vi "Delete.vi"(5 "Delete all found":bool, 6 "$Path or Item Name":string, 7 "error in (no error)":errorcluster, 9 "Offset":i32, 10 "JSON":string="{}") -> (0 "error out":errorcluster, 1 "<JSON> First Deleted Item":string, 2 "Number Deleted":i32, 3 "<JSON>":string caption="<JSON>With Item Deleted")   [LabVIEW 2021, in "json.facade.lvlib"]
doc: "Deletes JSON item at the JSON Path specified. If \"Delete all found\" is True, will delete all items matching the path. Else will just delete the first found."
uses:
  json.facade.lvlib
  jsontext/JSONtext.lvlib
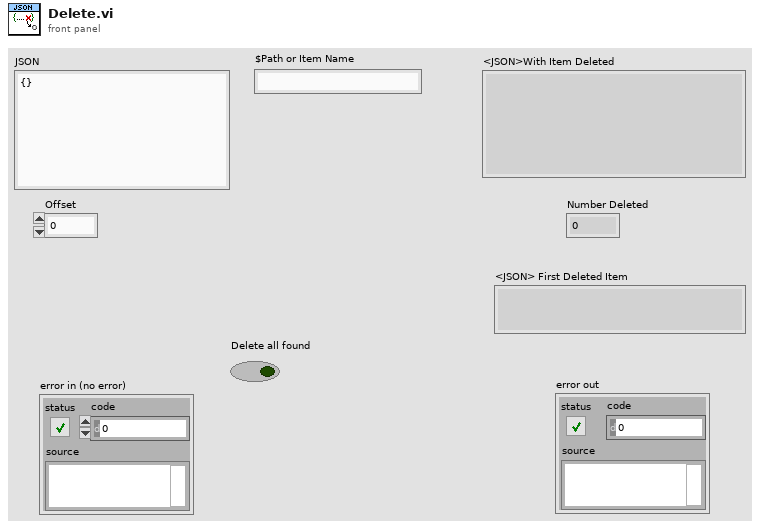
[diagram p1: front panel]
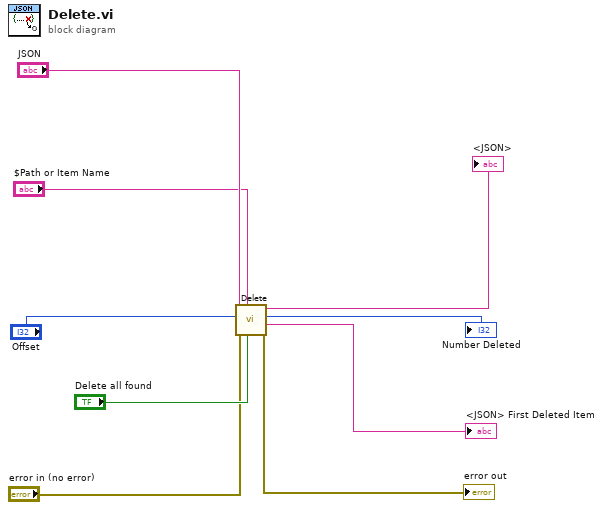
[diagram p0: block diagram]
diagram:
  n1 = call "Delete.vi"("Delete all found"="Delete all found", "$Path or Item Name"="$Path or Item Name", "error in (no error)"="error in (no error)", "Offset"="Offset", "JSON"="JSON") -> ("error out"=→"error out":errorcluster, "<JSON> First Deleted Item"=→"<JSON> First Deleted Item":string, "Number Deleted"=→"Number Deleted":i32, "<JSON>"=→"<JSON>":string)  [unwired: 2 in]
